vi "rp_arrange_diagram.vi"(6 "Variant in":variant, 7 "Shift Pressed?":bool, 8 "error in (no error)":errorcluster, 10 "QD Combo Box Ref":refnum<vi>, 11 "QD Launch VI Ref":refnum<vi>) -> (0 "error out":errorcluster, 4 "Variant out":variant)   [LabVIEW 2019]
doc: "Arranges the selected block diagram objects Left-to-Right or Right-to-Left. If nothing is selected, this arranges the control and indicator terminals to the connected terminals.\n\nCreated by: Ryan Pacini\n\nDefault Shortcut - [A]"
uses:
  _rp_support.llb/rp_arrange.ctl
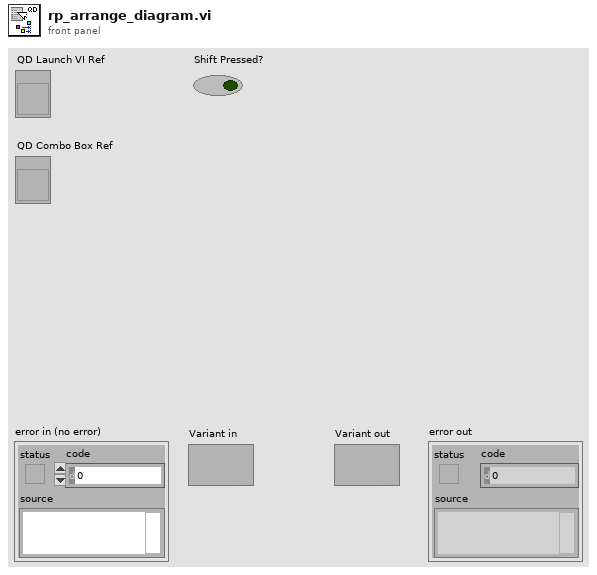
[diagram p1: front panel]
types:
  T1 = typedef "rp_arrange.ctl" = enum8{"left_to_right", "right_to_left"}
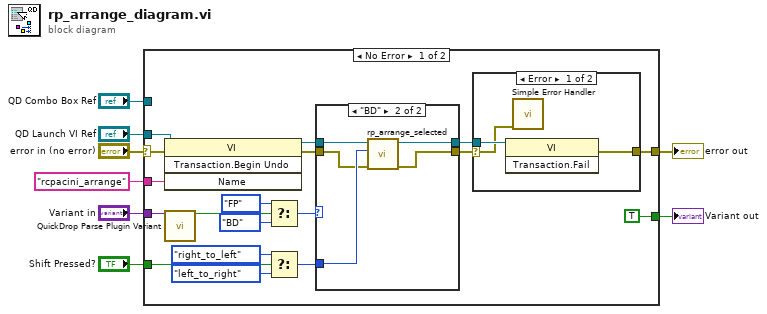
[diagram p0: block diagram]
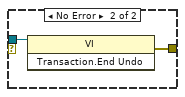
[diagram p3: hidden frame]
diagram:
  n1 = case shown="No Error" "error in (no error)" {
    selector: "error in (no error)" -> [w26 w39]
    tunnel: [w25 w39] -> w3
    tunnel: "QD Launch VI Ref" -> [w21 _]
    tunnel: "rcpacini_arrange" ("Undo Name") -> [w24 _]
    tunnel: "Variant in" -> [w22 _]
    tunnel: [TRUE _] -> w4
    tunnel: "QD Combo Box Ref" -> [_ _]
    tunnel: "Shift Pressed?" -> [w16 _]
    frame No Error {
      n2 = invoke class="VI" method="Transaction.Begin Undo"(reference=w21, error in=w26, "Name"=w24) -> (reference out=w20:refnum<vi>, error out=w19:errorcluster)  [unwired: 1 in, 2 out]
      n3 = call <vilib>:"QuickDrop Parse Plugin Variant.vi"("QDKS Variant in"=w22) -> ("QD Launch VI Panel?"=w12:bool)  [unwired: 12 in, 2 out]
      n4 = Select(t=enum8{"FP", "BD"}."FP" ("Panel"), s=w12, f=enum8{"FP", "BD"}."BD" ("Panel")) -> (s? t:f=w11:enum8{"FP", "BD"})
      n5 = Select(t=rp_arrange."right_to_left" ("Arrange"), s=w16, f=rp_arrange."left_to_right" ("Arrange")) -> (s? t:f=w15:T1)
      n6 = case shown="\"BD\"" w11 {
        tunnel: w20 -> [w28 w30]
        tunnel: w19 -> [w27 w29]
        tunnel: [w27 w33] -> w18
        tunnel: [w28 w32] -> w17
        tunnel: w15 -> [_ w31]
        frame "FP" {
        }
        frame "BD" {
          n7 = call "rp_arrange_selected.vi"("error in (no error)"=w29, "Arrange"=w31, "VI Refnum in"=w30) -> ("error out"=w33:errorcluster, "VI Refnum out"=w32:refnum<vi>)  [unwired: 7 in]
        }
      }
      n8 = case shown="Error" w18 {
        selector: w18 -> [w34 _]
        tunnel: w17 -> [w35 w37]
        tunnel: [w36 w38] -> w25
        frame Error {
          n9 = invoke class="VI" method="Transaction.Fail"(reference=w35) -> (error out=w36:errorcluster)  [unwired: 2 in, 2 out]
          n10 = call <vilib>:"Simple Error Handler.vi"("error in (no error)"=w34) -> ()  [unwired: 4 in, 5 out]
        }
        frame No Error {
          n11 = invoke class="VI" method="Transaction.End Undo"(reference=w37) -> (error out=w38:errorcluster)  [unwired: 2 in, 2 out]
        }
      }
    }
    frame Error {
    }
  }
  "error out" <- w3
  "Variant out" <- w4
